vi "Popup Menu Test Panel.vi"() -> ()   [LabVIEW 2020]
uses:
  <vilib>/Utility/miscctls.llb/LVPointTypeDef.ctl
panel:
  out "Error":errorcluster
  in  "Quit":bool
  in  "Text Input":string
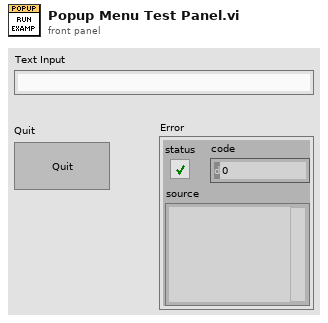
[diagram p1: front panel]
types:
  T1 = typedef "LVPointTypeDef.ctl" = cluster{"Horizontal":i16, "Vertical":i16}
  T2 = enum32{"Invalid", "Standard", "Closed", "Hidden", "Minimized", "Maximized"}
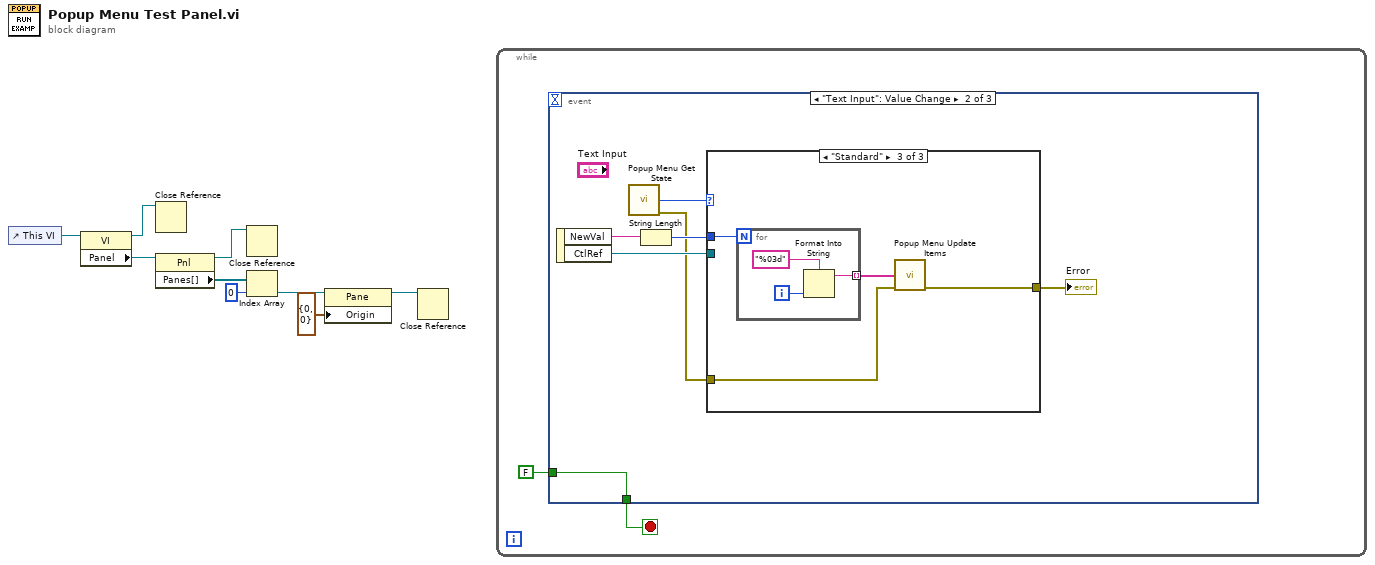
[diagram p0: block diagram]
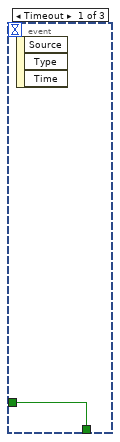
[diagram p2: hidden frame]
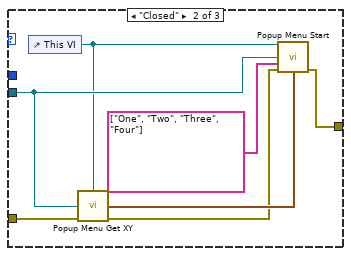
[diagram p4: hidden frame]
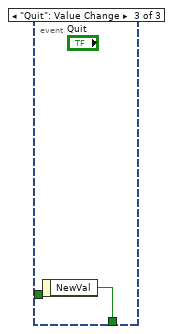
[diagram p5: hidden frame]
diagram:
  n1 = control-ref of="This VI"() -> (w9:refnum<vi>)
  n2 = property class="VI"(reference=w9) -> (reference out=w1:refnum<vi>, "Panel"=w8:refnum<vi>)  [unwired: 1 in, 1 out]
  n3 = Close Reference(reference=w1) -> ()  [unwired: 1 in, 1 out]
  n4 = property class="Pnl"(reference=w8) -> (reference out=w2:refnum<vi>, "Panes[]"=w7:refnum<vi>[])  [unwired: 1 in, 1 out]
  n5 = Close Reference(reference=w2) -> ()  [unwired: 1 in, 1 out]
  n6 = Index Array(array=w7, index=0) -> (element=w5:refnum<vi>)
  n7 = property class="Pane"(reference=w5, "Origin"=T1 {"Horizontal"=0, "Vertical"=0}) -> (reference out=w3:refnum<vi>)  [unwired: 1 in, 1 out]
  n8 = Close Reference(reference=w3) -> ()  [unwired: 1 in, 1 out]
  n9 = while {
    stop <- w10 stop-if-true
    n10 = event shown="[1] \"Text Input\": Value Change" {
      selector: _ -> [_ _ _]
      dyn-events: _ -> [_ _ _]
      timeout: _ -> [_ _ _]
      tunnel: FALSE -> [w12 w19 _]
      tunnel: [w12 w19 w35] -> w10
      event Timeout {
        n11 = event-data() -> ()  [unwired: 1 in, 3 out]
      }
      event "Text Input": Value Change {
        n12 = event-data() -> ("NewVal"=w18:string, "CtlRef"=w16:refnum<vi>)  [unwired: 1 in]
        n13 = call "Popup Menu Get State.vi"() -> ("FP State"=w15:T2, "Error Out"=w14:errorcluster)  [unwired: 14 in]
        n14 = String Length(string=w18) -> (length=w17:i32)
        n15 = case shown="\"Standard\"" w15 {
          tunnel: w17 -> [_ _ w30]
          tunnel: w16 -> [_ w27 _]
          tunnel: w14 -> [w20 w22 w29]
          tunnel: [w20 w21 w28] -> w13
          frame Default {
          }
          frame "Closed" {
            n16 = control-ref of="This VI"() -> (w26:refnum<vi>)
            n17 = call "Popup Menu Get XY.vi"("VI Ref"=w26, "Str Ctrl Ref"=w27, "Errror In"=w22) -> ("Screen Coordinates"=w25:T1, "Error Out"=w23:errorcluster)  [unwired: 11 in]
            n18 = call "Popup Menu Start.vi"("VI Ref"=w26, "Str Ctrl Ref"=w27, "Initial Menu Options"=string[] ["One", "Two", "Three", "Four"], "Error In"=w23, "XY Position"=w25) -> ("Error Out"=w21:errorcluster)  [unwired: 10 in]
          }
          frame "Standard" {
            n19 = for {
              N: w30 -> [_]
              tunnel: [w32] -> w31 mode=indexing
              i -> [w34]
              n20 = Format Into String(format string="%03d", w34) -> (resulting string=w32:string)  [unwired: 2 in, 1 out]
            }
            n21 = call "Popup Menu Update Items.vi"("Menu Items"=w31, "Error In"=w29) -> ("Error Out"=w28:errorcluster)  [unwired: 13 in]
          }
        }
        "Error" <- w13
      }
      event "Quit": Value Change {
        n22 = event-data() -> ("NewVal"=w35:bool)  [unwired: 1 in]
      }
    }
  }
